vi "Update Git Confirmation Window.vi"(8 "error in (no error)":errorcluster, 11 "Guardian Subpanel in":refnum<class "Guardian Subpanel.lvclass">) -> (3 "Guardian Subpanel out":refnum<class "Guardian Subpanel.lvclass">)   [LabVIEW 2026, in "TALOS.lvlib" / "Guardian Subpanel.lvlib" / "Guardian Subpanel.lvclass"]
uses:
  Guardian Subpanel.lvclass
  C:/LabVIEW Code/TALOS/talos/Father of all uServices/Father of all uServices/Father of all uServices.lvclass
  C:/LabVIEW Code/TALOS/builds/Actor Framework PPL/Actor Framework.lvlibp/1abvi3w/vi.lib/ActorFramework/Actor/Actor.lvclass
  Guardian/Guardian/Git Update Cluster.ctl
  Guardian/Guardian/Buttons_UI.ctl
  Guardian/Guardian Messages/Button Pressed Msg/Button Pressed Msg.lvclass/Button Pressed Msg.ctl
  builds/Actor Framework PPL/Actor Framework.lvlibp/1abvi3w/vi.lib/ActorFramework/Message Enqueuer/Message Priority.ctl
  Ancestor/Ancestor/Ancestor.lvclass/Ancestor.ctl
  Ancestor/Ancestor Messages/Process EH Error Msg/Process EH Error Msg.lvclass/Process EH Error Msg.ctl
  Support VIs/Generate Error.vi
  FGV/Error Memory/Get Error Description.vi
  Support VIs/Get PC name.vi
  Ancestor/Ancestor/Read ID.vi
  Support VIs/Get Class Name.vi
  <vilib>/Utility/error.llb/Clear Errors.vi
  FGV/Error Memory/Error Memory Core.vi
  <vilib>/AdvancedString/Delimited String to 1D String Array.vi
  <vilib>/AdvancedString/Delimited String to 1D String Array (string).vi
  Support VIs/Circus Root Path.vi
  FGV/Error Memory/Error Crt Lvl checker.vi
  FGV/Error Memory/Error Memory Core.vi/40c8088d-b597-4017-91af-faa98e00292e.vi
  FGV/Error Memory/Error Memory Core.vi/d4a3ab98-063c-4e44-b43d-fbdcfe6c2be2.vi
  builds/Actor Framework PPL/Actor Framework.lvlibp/1abvi3w/vi.lib/ActorFramework/Message Enqueuer/Enqueue.vi
  Support VIs/Global Memory.vi
  <vilib>/Utility/LVClass/Get LV Class Name.vi
  Support VIs/Is in Packed Library.vi
  Support VIs/TALOS Root path.vi
  Support VIs/Read CSV worksheet.vi
  Support VIs/Global Constants.vi
  <vilib>/Utility/error.llb/General Error Handler.vi
  Support VIs/Error Log.vi
  Guardian/Guardian Messages/Button Pressed Msg/Button Pressed Msg.lvclass
  Ancestor/Ancestor/Ancestor.lvclass
  <vilib>/Comparison/Equal/Equal Functor/Equal Functor.lvclass
  Ancestor/Ancestor Messages/Process EH Error Msg/Process EH Error Msg.lvclass
  builds/Actor Framework PPL/Actor Framework.lvlibp/1abvi3w/vi.lib/ActorFramework/Actor/Actor.lvclass
  builds/Actor Framework PPL/Actor Framework.lvlibp/1abvi3w/vi.lib/ActorFramework/Message Enqueuer/Message Enqueuer.lvclass
  TALOS.lvlib
  Guardian/Guardian/Guardian.lvclass
  Father of all uServices/Father of all uServices/Father of all uServices.lvclass
panel:
  in  "Cancel":bool
  in  "OK":bool
  out "Message":string
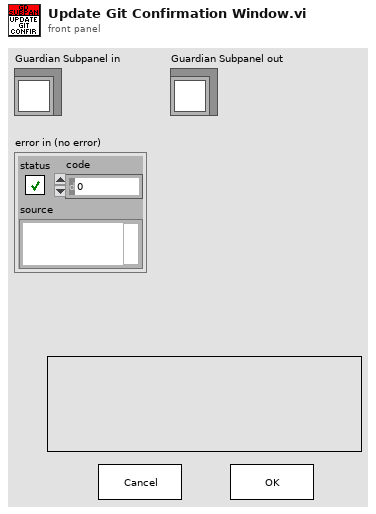
[diagram p1: front panel]
types:
  T1 = typedef "TALOS.lvlib/Guardian.lvlib/Guardian.lvclass/Git Update Cluster.ctl" = cluster{"branch name":string, "include critical PCs":bool, "update from git":bool}
  T2 = typedef "TALOS.lvlib/Guardian.lvlib/Guardian.lvclass/Buttons_UI.ctl" = enum16{"Start uService", "Kill uService", "Stop uService", "Stop", "Start online checks", "Stop online checks", "Send Pat to all GDs", "Reload INI files", "Update from GIT", "RUN", "Reset ABORT", "Check Bearer", "Send I Exist", "Change Run Config", "Add uSs from Config", "Realign uSs from Config", "Send Run Config to GD"}
  T3 = typedef "Actor Framework.lvlibp/Message Enqueuer.lvclass/Message Priority.ctl" = enum16{"Low", "Normal", "High"}
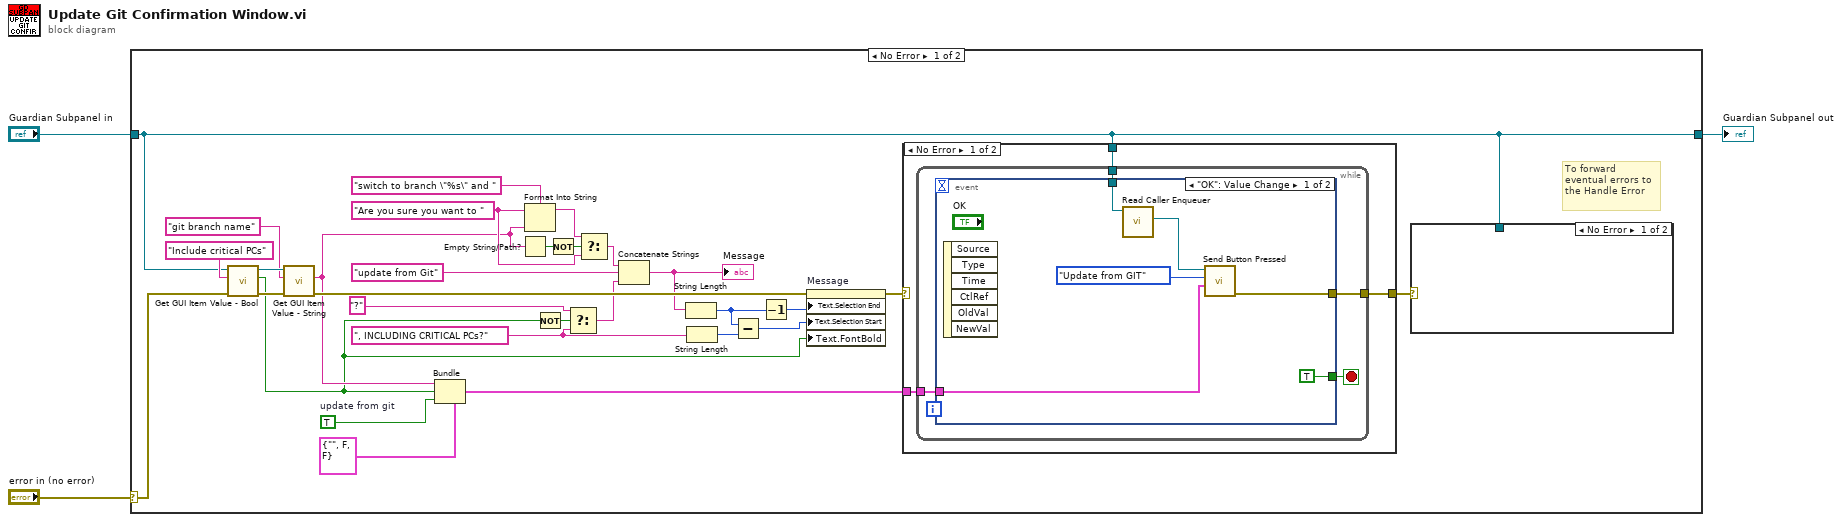
[diagram p0: block diagram]
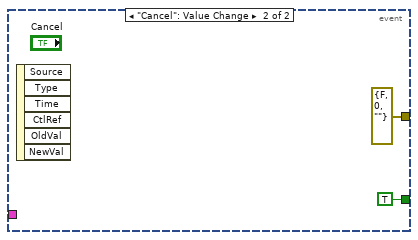
[diagram p2: hidden frame]
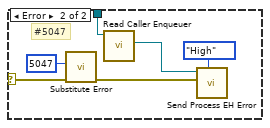
[diagram p4: hidden frame]
diagram:
  n1 = case shown="No Error" "error in (no error)" {
    selector: "error in (no error)" -> [w29 _]
    tunnel: [w30 w56] -> w1
    tunnel: "Guardian Subpanel in" -> [w30 w56]
    frame No Error {
      w4 = TRUE  # update from git
      w13 = ", INCLUDING CRITICAL PCs?"
      w9 = "Are you sure you want to "
      # "To forward eventual errors to the Handle Error"
      n2 = call "Get GUI Item Value - Bool.vi"("error in (no error)"=w29, "FP Item Name"="Include critical PCs", "uService Template in"=w30) -> ("error out"=w27:errorcluster, "Value"=w6:bool, "uService Template out"=w28:refnum<class "Guardian Subpanel.lvclass">)  [unwired: 6 in]
      n3 = call "Get GUI Item Value - String.vi"("error in (no error)"=w27, "FP Item Name"="git branch name", "uService Template in"=w28) -> ("error out"=w33:errorcluster, "Value"=w8:string)  [unwired: 6 in, 1 out]
      n4 = Bundle(cluster=T1 {"branch name"="", "include critical PCs"=FALSE, "update from git"=FALSE} ("output cluster"), "branch name"=w8, "include critical PCs"=w6, "update from git"=w4) -> (w25:T1)
      n5 = Empty String/Path?(string/path=w8) -> (empty?=w21:bool)
      n6 = Format Into String(format string="switch to branch \"%s\" and ", initial string=w9, w8) -> (resulting string=w19:string)  [unwired: 1 in, 1 out]
      n7 = Not(x=w6) -> (.not. x?=w16:bool)
      n8 = Not(x=w21) -> (.not. x?=w20:bool)
      n9 = Select(t="?" ("f"), s=w16, f=w13) -> (s? t:f=w17:string)
      n10 = Select(t=w19, s=w20, f=w9) -> (s? t:f=w18:string)
      n11 = Concatenate Strings(w18, "update from Git" ("string"), w17) -> (w22:string)
      "Message" <- w22
      n12 = String Length(string=w22) -> (length=w14:i32)
      n13 = String Length(string=w13) -> (length=w15:i32)
      n14 = Subtract(x=w14, y=w15) -> (x-y=w24:i32)
      n15 = Decrement(x=w14) -> (x-1=w23:i32)
      n16 = property on="Message" class="Str"(error in=w33, "Text.Selection End"=w23, "Text.Selection Start"=w24, "Text.FontBold"=w6) -> (error out=w7:errorcluster)  [unwired: 1 in, 1 out]
      n17 = case shown="No Error" w7 {
        selector: w7 -> [_ w49]
        tunnel: [w35 w49] -> w31
        tunnel: w30 -> [w36 _]
        tunnel: w25 -> [w34 _]
        frame No Error {
          n18 = while {
            tunnel: w36 -> [w39]
            tunnel: [w38] -> w35
            tunnel: w34 -> [w37]
            stop <- w40 stop-if-true
            n19 = event shown="[0] \"OK\": Value Change" {
              selector: _ -> [_ _]
              dyn-events: _ -> [_ _]
              timeout: _ -> [_ _]
              tunnel: [TRUE TRUE] -> w40
              tunnel: w39 -> [w43 _]
              tunnel: [w42 errorcluster {"status"=FALSE, "code"=0, "source"=""} ("error out")] -> w38
              tunnel: w37 -> [w41 _]
              event "OK": Value Change {
                n20 = event-data() -> ()  [unwired: 1 in, 6 out]
                n21 = call "Read Caller Enqueuer.vi"("Actor"=w43) -> ("Caller Enqueuer"=w44:refnum<class "Message Enqueuer.lvclass">)  [unwired: 10 in]
                n22 = call "Send Button Pressed.vi"("Data"=w41, "Button"=Buttons_UI."Update from GIT", "Message Enqueuer"=w44) -> ("error out"=w42:errorcluster)  [unwired: 7 in, 1 out]
              }
              event "Cancel": Value Change {
                n23 = event-data() -> ()  [unwired: 1 in, 6 out]
              }
            }
          }
        }
        frame Error {
        }
      }
      n24 = case shown="No Error" w31 {
        selector: w31 -> [_ w52]
        tunnel: w30 -> [_ w53]
        frame No Error {
        }
        frame Error {
          # "#5047"
          n25 = call "Substitute Error.vi"("error in (no error)"=w52, "Error Code"=5047) -> ("error out"=w51:errorcluster)  [unwired: 9 in]
          n26 = call "Read Caller Enqueuer.vi"("Actor"=w53) -> ("Caller Enqueuer"=w54:refnum<class "Message Enqueuer.lvclass">)  [unwired: 10 in]
          n27 = call "Send Process EH Error.vi"("Message Priority (Normal)"=Message_Priority."High", "Error to process"=w51, "Message Enqueuer"=w54) -> ()  [unwired: 7 in, 2 out]
        }
      }
    }
    frame Error {
    }
  }
  "Guardian Subpanel out" <- w1
